vi "ConfigCreateXMLHeader.vi"() -> (0 "XML Header":string)   [LabVIEW 2018, in "Config.lvlib"]
uses:
  Config.lvlib
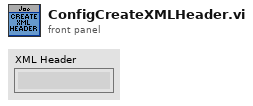
[diagram p1: front panel]
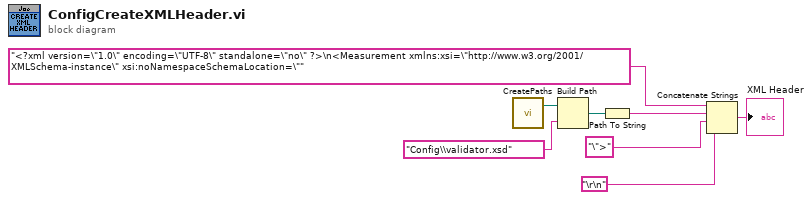
[diagram p0: block diagram]
diagram:
  n1 = call "CreatePaths.vi"() -> ("LibPath"=w4:path)  [unwired: 2 in, 1 out]
  n2 = Build Path(base path=w4, name or relative path="Config\\validator.xsd") -> (appended path=w3:path)
  n3 = Path To String(path=w3) -> (string=w2:string)
  n4 = Concatenate Strings("<?xml version=\"1.0\" encoding=\"UTF-8\" standalone=\"no\" ?>\n<Measurement xmlns:xsi=\"http://www.w3.org/2001/XMLSchema-instance\" xsi:noNamespaceSchemaLocation=\"", w2, "\">", "\r\n") -> (→"XML Header":string)
